vi "Main.vi"() -> ()   [LabVIEW 2014, in "4. Inheriting from a Widget.lvlib"]
doc: "This example takes the widget code from \"3a. Connecting a Signal to a Qt Slot\" and encapsulates it in a dedicated LVClass called \"Number Widget\".\n\nThere are a few reasons to do this:\n- To keep code organized. Notice that the block diagram for Main.vi is simpler in Example 4 than Example 3a.\n- To inherit the features of existing widgets, without having to rewriting it from scratch.\n- To make it easy to re-use your custom widget code. See tutorial \"6. Reusing Components Dynamically\".\n\n\n<b>Showcase</b>\n- Inheritable GUI components\n\n\nCopyright (c) 2019 Sze Howe Koh.\nThis code is licensed under the MIT license."
uses:
  4. Inheriting from a Widget.lvlib
  <vilib>/addons/LQ/LQ Core/QSize.ctl
  <vilib>/addons/LQ/Qt Widgets/QWidget/resize.vi
  <vilib>/addons/LQ/Qt Widgets/QWidget/setVisible.vi
  <vilib>/addons/LQ/LQ Core/LQCoreEngine/LQCoreEngine.lvclass
  Number Widget/Number Widget.lvclass
panel:
  in  "Stop Button":bool
  # "Prerequisite knowledge/experience\n- Examples 1-3 in this series\n- LabVIEW object-oriented programming (http://www.ni.com/white-paper/3573/en/)\n\n\nDescription\nThis example takes the widget code from 3a. Connecting a Signal to a Qt Slot and encapsulates it in a\ndedicated LVClass called Number Widget.\n\nThere are a few reasons to do this:\n- To keep code organized. Notice that the block diagram for Main.vi is simpler in Example 4 than in\n  Example 3a.\n- To inherit the features of existing widgets, without having to rewriting it from scratch.\n- To make it easy to re-use your custom widget code. See tutorial 6. Reusing Components Dynamically.\n\n\nShowcase\n- Inheritable GUI components"
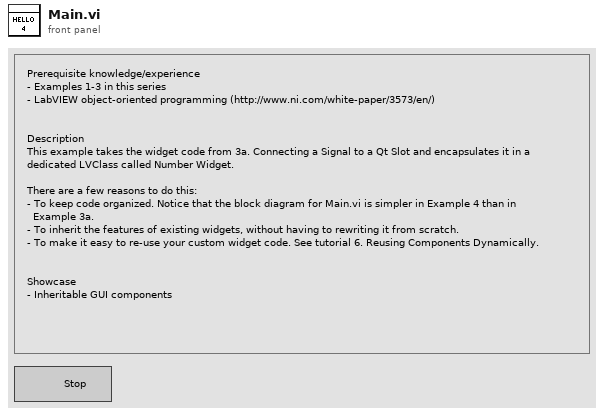
[diagram p1: front panel]
types:
  T1 = typedef "QSize.ctl" = cluster{"width":i32, "height":i32}
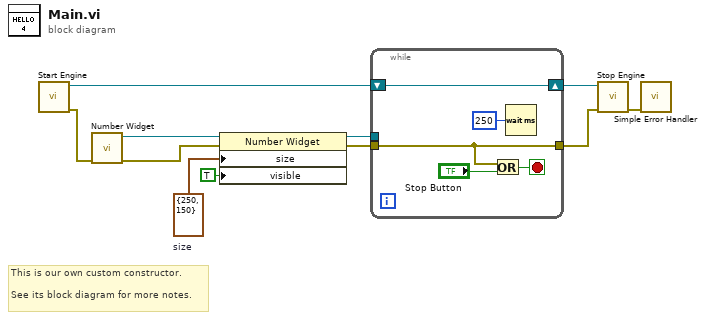
[diagram p0: block diagram]
diagram:
  w7 = T1 {"width"=250, "height"=150}  # size
  # "This is our own custom constructor.\n\nSee its block diagram for more notes."
  n1 = call <vilib>:"Start Engine.vi"() -> ("Error Out"=w2:errorcluster, "New Engine"=w11:refnum<class "LQCoreEngine.lvclass">)  [unwired: 10 in]
  n2 = call "Number Widget.vi"("Error In"=w2) -> ("Error Out"=w1:errorcluster, "New Number Widget"=w3:refnum<class "Number Widget.lvclass">)  [unwired: 9 in]
  n3 = property class="Number Widget"(reference=w3, error in=w1, "size"=w7, "visible"=TRUE) -> (reference out=w4:refnum<class "Number Widget.lvclass">, error out=w9:errorcluster)
  n4 = while {
    shift-right: [w16] -> w10
    shift-left: w11 -> [w16]
    tunnel: w9 -> [w12]
    tunnel: [w12] -> w5
    tunnel: w4 -> [_]
    stop <- w14 stop-if-true
    n5 = Or(x=w12, y="Stop Button") -> (x .or. y?=w14:bool)
    n6 = Wait (ms)(milliseconds to wait=u32 250) -> ()  [unwired: 1 out]
  }
  n7 = call <vilib>:"Stop Engine.vi"("Error In"=w5, "LQCoreEngine"=w10) -> ("Error Out"=w8:errorcluster)  [unwired: 9 in]
  n8 = call <vilib>:"Simple Error Handler.vi"("error in (no error)"=w8) -> ()  [unwired: 4 in, 5 out]
